vi "spot.XYG_1.1.vi"(0 "ArrayMask(X)":i32[](array[numeric])=[0, 1, 2, 3, 4, 5, 6, 7, 8, 9, 10, 11, 12, 13, 24, 25], 1 "fromX":dbl format="%.2f", 2 "toX":dbl format="%.2f", 3 "gussConvolution":bool, 4 "Th(streap)":dbl=3.0, 5 "fromY":dbl format="%.2f", 6 "toY":dbl format="%.2f", 7 "ArrayMask(Y )":i32[](array[numeric])=[0, 1, 2, 3, 4, 5, 6, 7, 8, 9, 10, 11, 12, 13, 24, 25], 8 "sigmaPed(x)":dbl[](array[numeric])=[0.0, 0.0, 0.0, 0.0, 0.0, 0.0, 0.0, 0.0, 0.0, 0.0, 0.0, 0.0, 0.0, 0.0, 0.0, 1.0] format="%.2f", 9 "sigmaPed(Y)":dbl[](array[numeric])=[0.0, 0.0, 0.0, 0.0, 0.0, 0.0, 0.0, 0.0, 0.0, 0.0, 0.0, 0.0, 0.0, 0.0, 0.0, 1.0] format="%.2f", 10 "Ped(x)":dbl[](array[numeric])=[0.0, 0.0, 0.0, 0.0, 0.0, 0.0, 0.0, 0.0, 0.0, 0.0, 0.0, 0.0, 0.0, 0.0, 0.0, 0.0] format="%.2f", 11 "Ped(Y)":dbl[](array[numeric])=[0.0, 0.0, 0.0, 0.0, 0.0, 0.0, 0.0, 0.0, 0.0, 0.0, 0.0, 0.0, 0.0, 0.0, 0.0, 0.0] format="%.2f", 12 "init?":bool, 13 "dataRaw":dbl[](array[numeric]) format="%.2f", 14 "odo/sili":bool, 15 "STREAP":i32[](array[numeric]), 16 "1/2":bool) -> (20 "Y plot":cluster{cluster{ext, ext}[]}[](graph), 21 "mean Y":dbl format="%.2f", 22 "sigma Y":dbl format="%.2f", 25 "mean X":dbl format="%.2f", 26 "sigmaX":dbl format="%.2f", 27 "X plot":cluster{cluster{ext, ext}[]}[](graph))   [LabVIEW 2014]
panel:
  out "dataOut":dbl[](array[numeric]) format="%.2f"
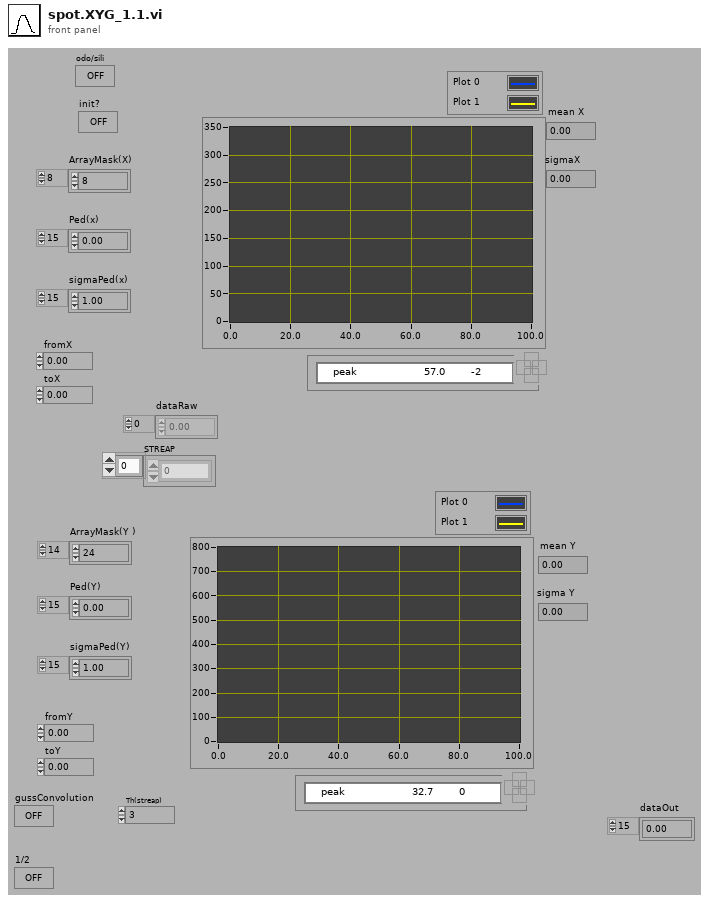
[diagram p1: front panel]
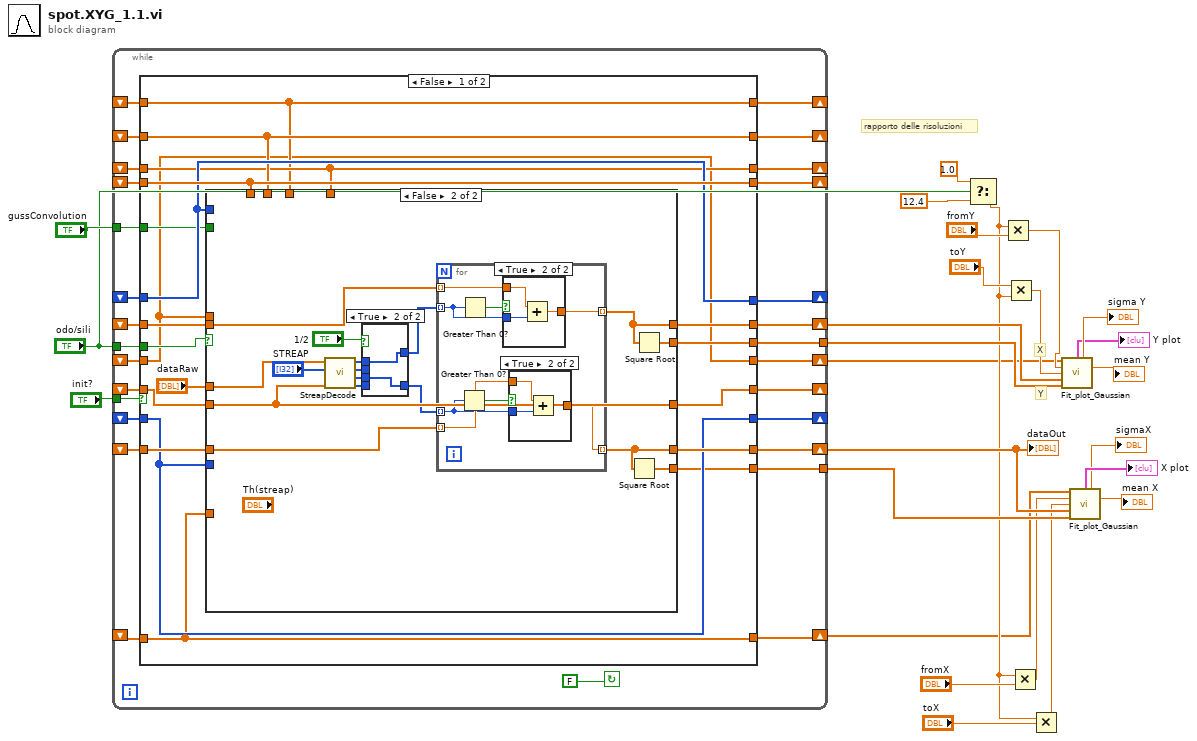
[diagram p0: block diagram]
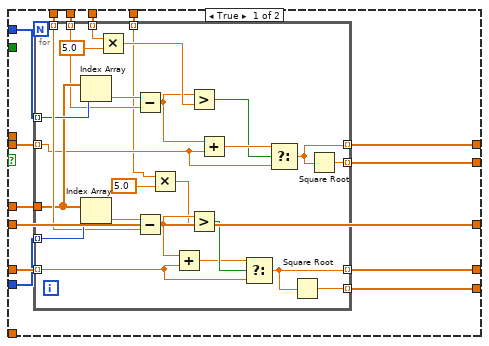
[diagram p2: hidden frame]
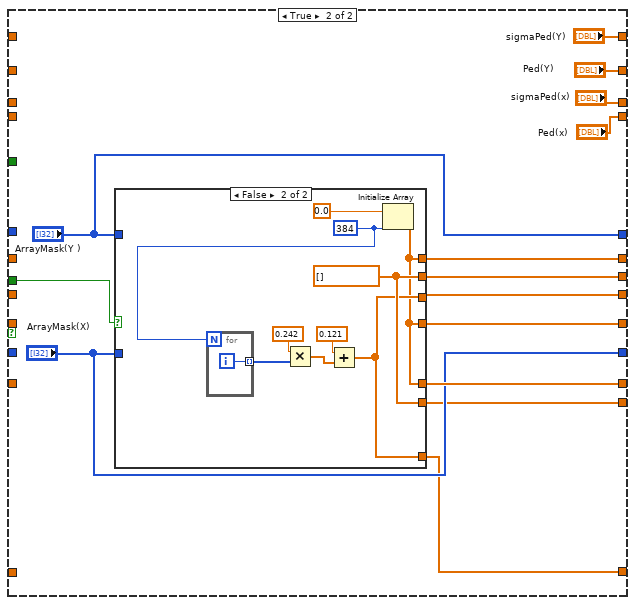
[diagram p6: hidden frame]
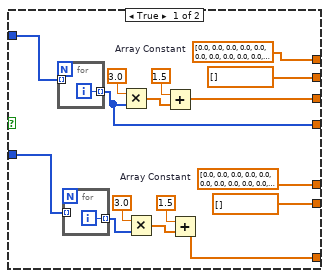
[diagram p7: hidden frame]
diagram:
  # "rapporto delle risoluzioni"
  # "Y"
  # "X"
  n1 = while {
    tunnel: [w43] -> w23
    shift-left: _ -> [w44]
    shift-right: [w45] -> w1
    shift-left: _ -> [w46]
    shift-right: [w51] -> _
    shift-left: _ -> [w47]
    shift-right: [w50] -> _
    shift-left: _ -> [w48]
    shift-right: [w49] -> _
    tunnel: "init?" -> [w54]
    shift-left: _ -> [w52]
    shift-right: [w53] -> w24
    shift-right: [w40] -> _
    shift-left: _ -> [w37]
    shift-right: [w39] -> w14
    shift-left: _ -> [w35]
    shift-right: [w41] -> w2
    shift-left: _ -> [w36]
    tunnel: [w38] -> w15
    shift-right: [w34] -> _
    shift-left: _ -> [w32]
    shift-right: [w33] -> _
    shift-left: _ -> [w31]
    tunnel: "odo/sili" -> [w30]
    tunnel: "gussConvolution" -> [w29]
    shift-right: [w28] -> _
    shift-left: _ -> [w27]
    stop <- FALSE continue-if-true
    n2 = case shown="False" w54 {
      tunnel: [w71 w162] -> w53
      tunnel: w52 -> [w72 _]
      tunnel: [w62 "sigmaPed(x)"] -> w51
      tunnel: [w69 "Ped(x)"] -> w50
      tunnel: [w70 "ArrayMask(X)"] -> w49
      tunnel: w48 -> [w70 _]
      tunnel: w47 -> [w69 _]
      tunnel: w46 -> [w62 _]
      tunnel: [w57 w157] -> w45
      tunnel: w44 -> [w57 _]
      tunnel: [w68 w158] -> w43
      tunnel: [w64 "ArrayMask(Y )"] -> w40
      tunnel: [w58 w155] -> w41
      tunnel: [w66 w154] -> w39
      tunnel: [w65 w153] -> w38
      tunnel: w37 -> [w64 _]
      tunnel: w36 -> [w58 _]
      tunnel: w35 -> [w67 _]
      tunnel: [w61 "sigmaPed(Y)"] -> w34
      tunnel: [w63 "Ped(Y)"] -> w33
      tunnel: w32 -> [w61 _]
      tunnel: w31 -> [w63 _]
      tunnel: w30 -> [w60 w150]
      tunnel: w29 -> [w59 _]
      tunnel: [w55 w149] -> w28
      tunnel: w27 -> [w56 _]
      frame False {
        n3 = case shown="False" w60 {
          tunnel: "dataRaw" -> [w87 w126]
          tunnel: w72 -> [w86 w121]
          tunnel: [w85 w120] -> w71
          tunnel: w70 -> [w84 _]
          tunnel: w69 -> [w83 _]
          tunnel: [w82 w128] -> w68
          tunnel: w67 -> [w81 w123]
          tunnel: [w80 w122] -> w66
          tunnel: [w79 w127] -> w65
          tunnel: w64 -> [w78 _]
          tunnel: w63 -> [w77 _]
          tunnel: w62 -> [w76 _]
          tunnel: w61 -> [w75 _]
          tunnel: w59 -> [_ _]
          tunnel: w58 -> [_ _]
          tunnel: w57 -> [_ _]
          tunnel: w56 -> [w74 w124]
          tunnel: [w74 w124] -> w55
          frame True {
            n4 = for {
              tunnel: w84 -> [w112] mode=indexing
              tunnel: w87 -> [w98]
              tunnel: w83 -> [w100] mode=indexing
              tunnel: w75 -> [w110] mode=indexing
              tunnel: w86 -> [w107] mode=indexing
              tunnel: [w104] -> w85 mode=indexing
              tunnel: [w103] -> w82 mode=indexing
              tunnel: w78 -> [w99] mode=indexing
              tunnel: w81 -> [w95] mode=indexing
              tunnel: [w93] -> w80 mode=indexing
              tunnel: [w92] -> w79 mode=indexing
              tunnel: w77 -> [w91] mode=indexing
              tunnel: w76 -> [w89] mode=indexing
              n5 = Index Array(array=w98, index=w99) -> (element=w102:dbl)
              n6 = Index Array(array=w98, index=w112) -> (element=w111:dbl)
              n7 = Multiply(x=w110, y=5.0) -> (x*y=w101:dbl)
              n8 = Subtract(x=w102, y=w91) -> (x-y=w96:dbl)
              n9 = Subtract(x=w111, y=w100) -> (x-y=w106:dbl)
              n10 = Multiply(x=w89, y=5.0) -> (x*y=w88:dbl)
              n11 = Add(x=w106, y=w107) -> (x+y=w105:dbl)
              n12 = Greater?(x=w96, y=w101) -> (0:w94:bool)
              n13 = Greater?(x=w106, y=w88) -> (0:w108:bool)
              n14 = Add(x=w96, y=w95) -> (x+y=w97:dbl)
              n15 = Select(t=w105, s=w108, f=w107) -> (s? t:f=w104:dbl)
              n16 = Select(t=w97, s=w94, f=w95) -> (s? t:f=w93:dbl)
              n17 = Square Root(x=w104) -> (sqrt(x)=w103:dbl)
              n18 = Square Root(x=w93) -> (sqrt(x)=w92:dbl)
            }
          }
          frame False {
            n19 = call "StreapDecode.vi"("EmptyDataIn"=w124, "STREAP"="STREAP", "VALUE"=w126) -> ("X2"=w116:i32[], "X1"=w117:i32[], "Y2"=w113:i32[], "Y1"=w114:i32[])  [unwired: 1 in]
            n20 = case shown="True" "1/2" {
              tunnel: [w129 w131] -> w118
              tunnel: w117 -> [_ w132]
              tunnel: w116 -> [w130 _]
              tunnel: [w130 w132] -> w115
              tunnel: w114 -> [_ w131]
              tunnel: w113 -> [w129 _]
              frame False {
              }
              frame True {
              }
            }
            n21 = for {
              tunnel: w123 -> [w139] mode=indexing
              tunnel: w118 -> [w138] mode=indexing
              tunnel: [w137] -> w122 mode=indexing
              tunnel: w121 -> [w136] mode=indexing
              tunnel: w115 -> [w134] mode=indexing
              tunnel: [w135] -> w120 mode=indexing
              n22 = Greater Than 0?(x=w134) -> (x > 0?=w133:bool)
              n23 = Greater Than 0?(x=w138) -> (x > 0?=w140:bool)
              n24 = case shown="True" w140 {
                tunnel: w139 -> [w145 w148]
                tunnel: w138 -> [_ w147]
                tunnel: [w145 w146] -> w137
                frame False {
                }
                frame True {
                  n25 = Add(x=w148, y=w147) -> (x+y=w146:dbl)
                }
              }
              n26 = case shown="True" w133 {
                tunnel: w136 -> [w141 w144]
                tunnel: w134 -> [_ w143]
                tunnel: [w141 w142] -> w135
                frame False {
                }
                frame True {
                  n27 = Add(x=w144, y=w143) -> (x+y=w142:dbl)
                }
              }
            }
            n28 = Square Root(x=w120) -> (sqrt(x)=w128:dbl[])
            n29 = Square Root(x=w122) -> (sqrt(x)=w127:dbl[])
          }
        }
      }
      frame True {
        n30 = case shown="False" w150 {
          tunnel: [w178 w181] -> w162
          tunnel: "ArrayMask(X)" -> [w177 _]
          tunnel: [dbl[] [] w188] -> w158
          tunnel: [w173 w183] -> w157
          tunnel: "ArrayMask(Y )" -> [w167 _]
          tunnel: [w166 w183] -> w155
          tunnel: [w165 w181] -> w154
          tunnel: [dbl[] [] w188] -> w153
          tunnel: [w163 w181] -> w149
          frame True {
            w165 = dbl[] [0.0, 0.0, 0.0, 0.0, 0.0, 0.0, 0.0, 0.0, 0.0, 0.0, 0.0, 0.0, 0.0, 0.0, 0.0, 0.0]  # Array Constant
            w178 = dbl[] [0.0, 0.0, 0.0, 0.0, 0.0, 0.0, 0.0, 0.0, 0.0, 0.0, 0.0, 0.0, 0.0, 0.0, 0.0, 0.0]  # Array Constant
            n31 = for {
              tunnel: [w179] -> w163 mode=indexing
              tunnel: w167 -> [_] mode=indexing
              i -> [w179]
            }
            n32 = for {
              tunnel: w177 -> [_] mode=indexing
              tunnel: [w180] -> w174 mode=indexing
              i -> [w180]
            }
            n33 = Multiply(x=3.0, y=w163) -> (x*y=w169:dbl[])
            n34 = Multiply(x=3.0, y=w174) -> (x*y=w172:dbl[])
            n35 = Add(x=1.5, y=w169) -> (x+y=w166:dbl[])
            n36 = Add(x=1.5, y=w172) -> (x+y=w173:dbl[])
          }
          frame False {
            w187 = 384 ("index")
            w188 = dbl[] []
            n37 = for {
              N: w187 -> [_]
              tunnel: [w190] -> w182 mode=indexing
              i -> [w190]
            }
            n38 = Multiply(x=0.242, y=w182) -> (x*y=w185:dbl[])
            n39 = Add(x=0.121, y=w185) -> (x+y=w183:dbl[])
            n40 = Initialize Array(0.0, w187) -> (w181:dbl[])
          }
        }
      }
    }
  }
  "dataOut" <- w24
  n41 = Select(t=1.0 ("x"), s="odo/sili", f=12.4 ("x")) -> (s? t:f=w4:dbl)
  n42 = Multiply(x=w4, y="fromY") -> (x*y=w12:dbl)
  n43 = Multiply(x="toY", y=w4) -> (x*y=w11:dbl)
  n44 = Multiply(x=w4, y="fromX") -> (x*y=w8:dbl)
  n45 = Multiply(x=w4, y="toX") -> (x*y=w9:dbl)
  n46 = call "Fit_plot_Gaussian.vi"("X"=w2, "from"=w12, "to"=w11, "Y"=w14, "DY"=w15) -> (2:→"Y plot":cluster{cluster{ext, ext}[]}[], "sigma"=→"sigma Y":dbl, "m"=→"mean Y":dbl)  [unwired: 2 in, 6 out]
  n47 = call "Fit_plot_Gaussian.vi"("X"=w1, "from"=w8, "to"=w9, "Y"=w24, "DY"=w23) -> (2:→"X plot":cluster{cluster{ext, ext}[]}[], "sigma"=→"sigmaX":dbl, "m"=→"mean X":dbl)  [unwired: 2 in, 6 out]
